vi "Agilent PWM Preset.vi"(8 "error in (no error)":errorcluster, 11 "VISA Resource Name":refnum<visa-resource-name>) -> (0 "error out":errorcluster, 3 "dup VISA Resource Name":refnum<visa-resource-name>)   [LabVIEW 2011]
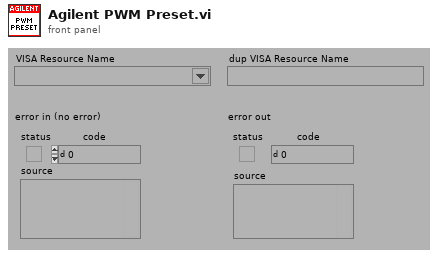
[diagram p1: front panel]
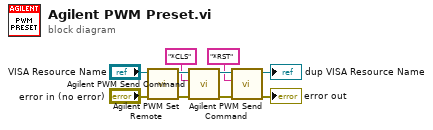
[diagram p0: block diagram]
diagram:
  n1 = call "Agilent PWM Set Remote.vi"("error in (no error)"="error in (no error)", "VISA Resource Name"="VISA Resource Name") -> ("error out"=w8:errorcluster, "dup VISA Resource Name"=w9:refnum<visa-resource-name>)  [unwired: 8 out]
  n2 = call "Agilent PWM Send Command.vi"("error in (no error)"=w8, "Command"="*CLS", "VISA Resource Name"=w9) -> ("error out"=w5:errorcluster, "dup VISA Resource Name"=w6:refnum<visa-resource-name>)  [unwired: 2 in, 5 out]
  n3 = call "Agilent PWM Send Command.vi"("error in (no error)"=w5, "Command"="*RST", "VISA Resource Name"=w6) -> ("error out"=→"error out":errorcluster, "dup VISA Resource Name"=→"dup VISA Resource Name":refnum<visa-resource-name>)  [unwired: 2 in, 5 out]
